vi "Set ICommunicate.vi"(10 "ICommunicate":refnum<class "ICommunicate.lvclass">, 11 "DBCCommunication in":refnum<class "DBC Communication.lvclass">) -> (3 "DBCCommunication out":refnum<class "DBC Communication.lvclass">)   [LabVIEW 2024, in "DBC Communication.lvclass"]
uses:
  DBC Communication.lvclass
  Interfaces/ICommunicate/ICommunicate.lvclass
  DBC Communication.lvclass/DBC Communication.ctl
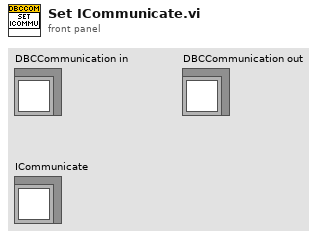
[diagram p1: front panel]
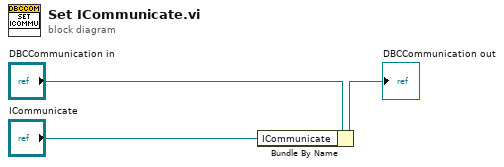
[diagram p0: block diagram]
diagram:
  n1 = Bundle By Name(cluster="DBCCommunication in", "ICommunicate"="ICommunicate") -> (→"DBCCommunication out":refnum<class "DBC Communication.lvclass">)
